vi "Release Child.vi"(8 "error in (no error)":errorcluster, 10 "Child HWID":u32, 11 "LV MDI in":refnum<class "LV MDI.lvclass">) -> (0 "error out":errorcluster, 3 "LV MDI out":refnum<class "LV MDI.lvclass">)   [LabVIEW 2016, in "LV MDI.lvclass"]
uses:
  LV MDI.lvclass
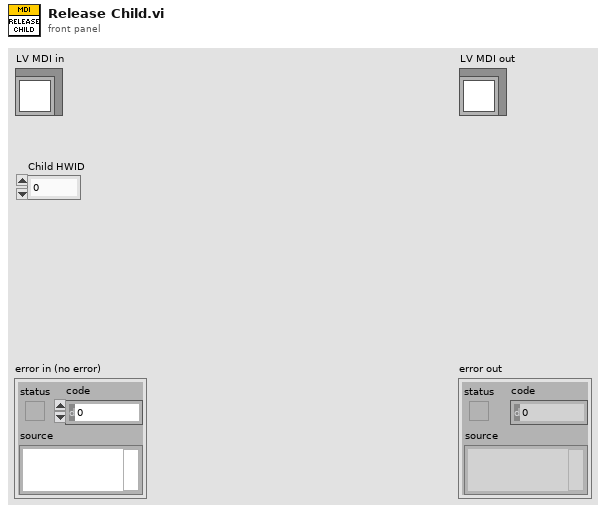
[diagram p1: front panel]
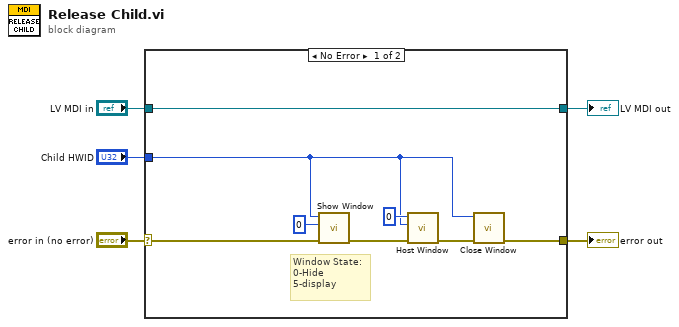
[diagram p0: block diagram]
diagram:
  n1 = case shown="No Error" "error in (no error)" {
    selector: "error in (no error)" -> [w10 w15]
    tunnel: [w12 w15] -> w4
    tunnel: [w13 w14] -> w2
    tunnel: "LV MDI in" -> [w13 w14]
    tunnel: "Child HWID" -> [w6 _]
    frame No Error {
      # "Window State:\n0-Hide\n5-display"
      n2 = call "Show Window.vi"("error in (no error)"=w10, "Window State"=u32 0, "hwnd"=w6) -> ("error out"=w8:errorcluster)  [unwired: 7 in, 1 out]
      n3 = call "Host Window.vi"("error in (no error)"=w8, "Child Hwnd"=w6, "Parent Hwnd"=0) -> ("error out"=w7:errorcluster)  [unwired: 8 in]
      n4 = call "Close Window.vi"("error in (no error)"=w7, "HWND"=w6) -> ("error out"=w12:errorcluster)  [unwired: 9 in]
    }
    frame Error {
    }
  }
  "error out" <- w4
  "LV MDI out" <- w2
